vi "Close.vi"(8 "error in (no error)":errorcluster, 11 "SLSC Switch in":refnum<class "SLSC Switch.lvclass">) -> (0 "error out":errorcluster)   [LabVIEW 2017, in "SLSC Switch.lvlib" / "SLSC Switch.lvclass"]
doc: "Disconnects all channels and terminates the SLSC-SWITCH session and all of its attributes and deallocates any memory resources the driver uses."
uses:
  SLSC Switch.lvclass
  SLSC Switch.lvclass/SLSC Switch.ctl
  <vilib>/National Instruments/SLSC Local or Remote Interface/SLSC Interface Class/SLSC Interface.lvclass
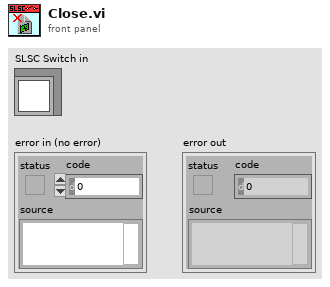
[diagram p1: front panel]
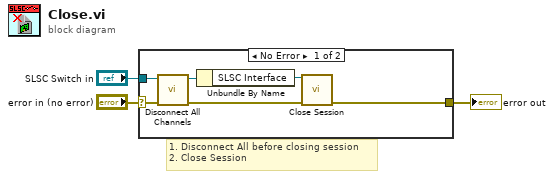
[diagram p0: block diagram]
diagram:
  # "1. Disconnect All before closing session\n2. Close Session"
  n1 = case shown="No Error" "error in (no error)" {
    selector: "error in (no error)" -> [w9 w10]
    tunnel: [w4 w10] -> w2
    tunnel: "SLSC Switch in" -> [w8 _]
    frame No Error {
      n2 = call "Disconnect All Channels.vi"("error in (no error)"=w9, "SLSC Switch in"=w8) -> ("error out"=w5:errorcluster, "SLSC Switch out"=w7:refnum<class "SLSC Switch.lvclass">)  [unwired: 8 in]
      n3 = Unbundle By Name(w7) -> ("SLSC Interface"=w6:refnum<class "SLSC Interface.lvclass">)
      n4 = call-dynamic "Close Session.vi"("SLSC Interface in"=w6, "error in (no error)"=w5) -> ("error out"=w4:errorcluster)  [unwired: 13 in]
    }
    frame Error {
    }
  }
  "error out" <- w2
